vi "3个数比大小--子程序·.vi"() -> ()   [LabVIEW 2017]
panel:
  out "C":dbl
  out "B":dbl
  out "A":dbl
  in  "c":dbl
  in  "b":dbl
  in  "a":dbl
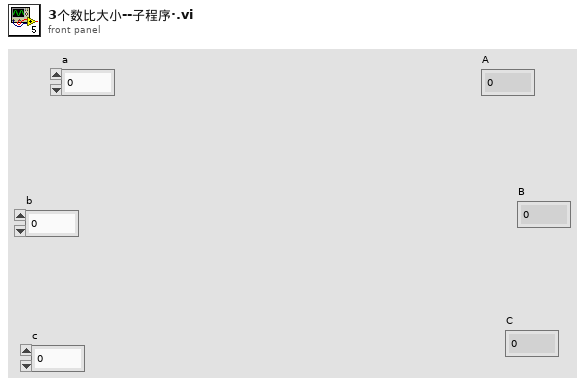
[diagram p1: front panel]
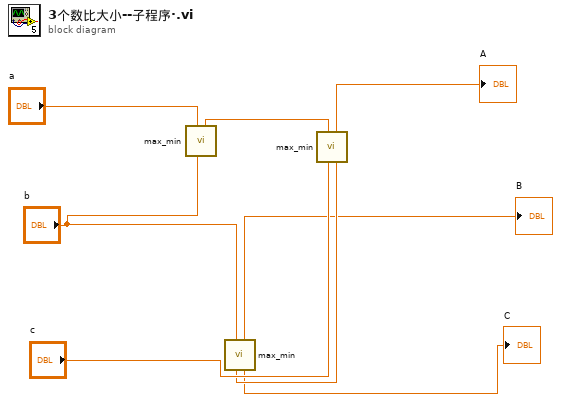
[diagram p0: block diagram]
diagram:
  n1 = call "max_min.vi"("b"="b", "a"="a") -> ("max"=w6:dbl)  [unwired: 8 in, 1 out]
  n2 = call "max_min.vi"("b"="c", "a"=w6) -> ("min"=w3:dbl, "max"=→"A":dbl)  [unwired: 8 in]
  n3 = call "max_min.vi"("b"=w3, "a"="b") -> ("min"=→"C":dbl, "max"=→"B":dbl)  [unwired: 8 in]
